vi "Link XML Start Tags with End Tags.vi"(8 "error in (no error)":errorcluster, 11 "xml in":T1) -> (0 "error out":errorcluster, 3 "xml out":T1)   [LabVIEW 2011]
uses:
  XML Structure - Cluster.ctl
  XML Tag Type - Enum.ctl
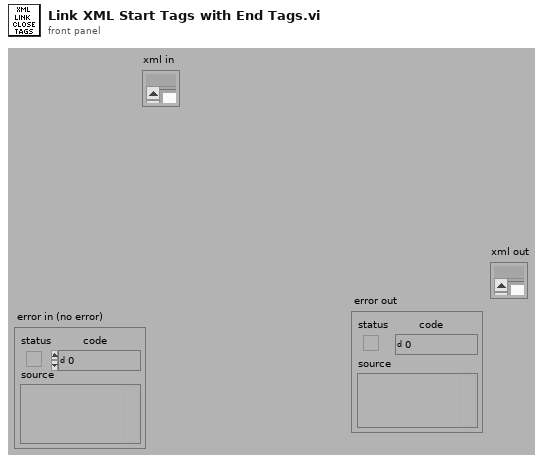
[diagram p1: front panel]
types:
  T1 = typedef "XML Structure - Cluster.ctl" = cluster{"tags":string[], "tag names":string[], "tag type":T2[], "offset":i32[], "close tag index":i32[], "xml":string, "Children":cluster{"children":i32[]}[], "parent index":i32[]}
  T2 = typedef "XML Tag Type - Enum.ctl" = enum16{"start tag", "empty tag", "end tag"}
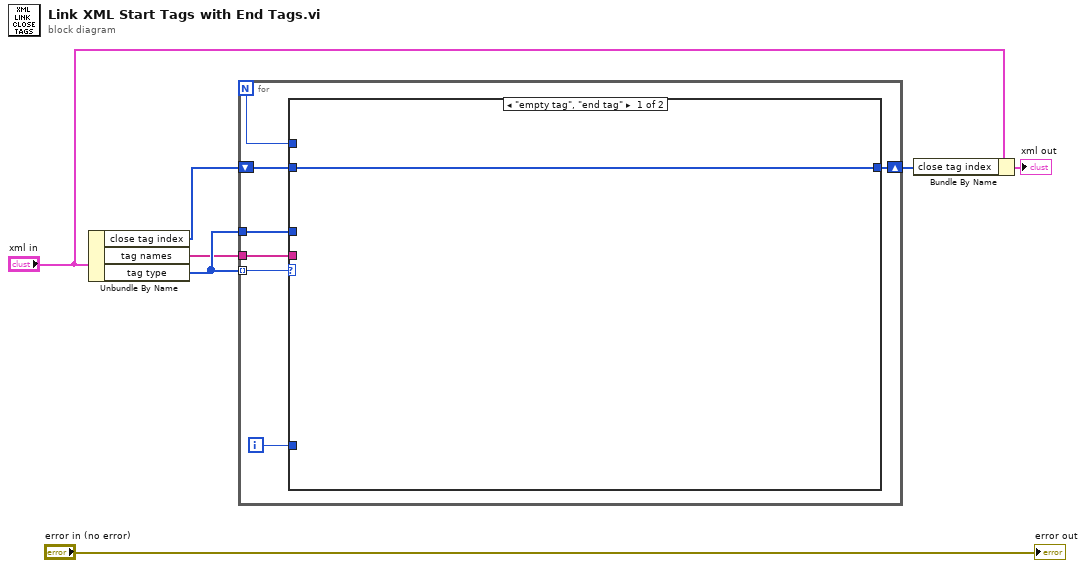
[diagram p0: block diagram]
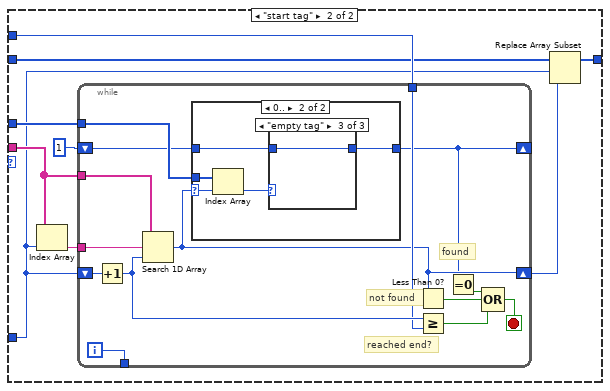
[diagram p2: hidden frame]
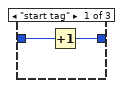
[diagram p4: hidden frame]
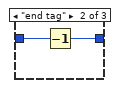
[diagram p5: hidden frame]
diagram:
  n1 = Unbundle By Name("xml in") -> ("close tag index"=w4:i32[], "tag names"=w2:string[], "tag type"=w3:T2[])
  n2 = for {
    N -> [w12]
    tunnel: w2 -> [w13]
    tunnel: w3 -> [w11] mode=indexing
    tunnel: w3 -> [w10]
    shift-right: [w8] -> w6
    shift-left: w4 -> [w9]
    i -> [w14]
    n3 = case shown="\"empty tag\", \"end tag\"" w11 {
      tunnel: w14 -> [_ w17]
      tunnel: w13 -> [_ w23]
      tunnel: w12 -> [_ w22]
      tunnel: w10 -> [_ w20]
      tunnel: w9 -> [w15 w19]
      tunnel: [w15 w18] -> w8
      frame "empty tag", "end tag" {
      }
      frame "start tag" {
        n4 = Index Array(array=w23, index=w17) -> (element=w24:string)
        n5 = while {
          tunnel: w24 -> [w31]
          tunnel: w23 -> [w38]
          shift-right: [w29] -> w16
          shift-left: w17 -> [w37]
          tunnel: w22 -> [w35]
          shift-right: [w26] -> _
          shift-left: 1 -> [w27]
          tunnel: w20 -> [w28]
          tunnel: [w25] -> _
          i -> [w25]
          stop <- w32 stop-if-true
          # "found"
          # "not found"
          # "reached end?"
          n6 = Increment(x=w37) -> (x+1=w36:i32)
          n7 = Search 1D Array(1D array=w38, element=w31, start index (0)=w36) -> (index of element=w29:i32)
          n8 = case shown="0.." w29 {
            selector: w29 -> [_ w44]
            tunnel: w28 -> [_ w43]
            tunnel: w27 -> [w39 w40]
            tunnel: [w39 w41] -> w26
            frame Default {
            }
            frame 0.. {
              n9 = Index Array(array=w43, index=w44) -> (element=w42:T2)
              n10 = case shown="\"empty tag\"" w42 {
                tunnel: [w45 w47 w49] -> w41
                tunnel: w40 -> [w46 w48 w49]
                frame "start tag" {
                  n11 = Increment(x=w46) -> (x+1=w45:i32)
                }
                frame "end tag" {
                  n12 = Decrement(x=w48) -> (x-1=w47:i32)
                }
                frame "empty tag" {
                }
              }
            }
          }
          n13 = Less Than 0?(x=w29) -> (x < 0?=w34:bool)
          n14 = Greater Or Equal?(x=w36, y=w35) -> (x >= y?=w33:bool)
          n15 = Equal To 0?(x=w26) -> (x = 0?=w30:bool)
          n16 = Compound Arithmetic op=OR(w30, w34, w33) -> (w32:bool)
        }
        n17 = Replace Array Subset(array=w19, new element=w16, index=w17) -> (w18:i32[])
      }
    }
  }
  n18 = Bundle By Name(cluster="xml in", "close tag index"=w6) -> (→"xml out":T1)
  "error out" <- "error in (no error)"
